vi "Test Pre-arm.vi"() -> ()   [LabVIEW 2021]
uses:
  Instruments/Lockin Digitizer Driver/Lockin Digitizer Configuration.ctl
  DAQmx Lockin Digitizer Driver.lvclass
  C:/GitHub/NHMFL_Core/Libraries/Instruments/Pulse Driver/Lockin Digitizer Driver/Lockin Digitizer Driver.lvclass
panel:
  out "error out":errorcluster
  out "DAQmx Lockin Digitizer Driver out":refnum<class "DAQmx Lockin Digitizer Driver.lvclass">
  in  "DAQmx Lockin Digitizer Driver in":refnum<class "DAQmx Lockin Digitizer Driver.lvclass">
  in  "Lockin Digitizer Configuration":T1={"Post-trigger delay"=0.01, "Post-trigger duration"=0.1, "Rate"=1000000.0, "Ranges"=[10.0], "Re-name channels"=["Bdor", "Idot", "V1", "V2", "I1", "I2", "I3"], "Active channels"="0:6", "External\nclock"=FALSE, "Frequencies"=[1.0, 2.0], "Time\nconstant"=1.0, "Output \namplitudes"=[1.0, 3.0], "Input\nchannles"=["2:3", "4:6"]} {"Output \namplitudes" format="%#_6pV"; "Time\nconstant" format="%#_6ps"; "Frequencies" format="%#_6pHz"; "Rate" format="%#_8pHz"; "Post-trigger duration" format="%#_6ps"; "Post-trigger delay" format="%#_6ps"; "Ranges" format="%#_6pV"}
  # "Digitizer config"
  # "Lock-in config"
  # "#0\n\n#1"
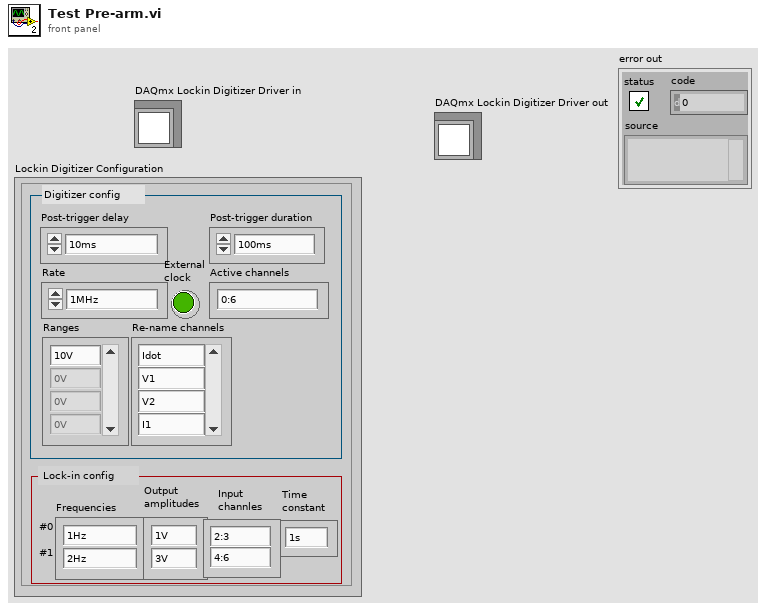
[diagram p1: front panel]
types:
  T1 = typedef "Lockin Digitizer Configuration.ctl" = cluster{"Post-trigger delay":dbl, "Post-trigger duration":dbl, "Rate":dbl, "Ranges":dbl[], "Re-name channels":string[], "Active channels":string, "External\nclock":bool, "Frequencies":dbl[], "Time\nconstant":dbl, "Output \namplitudes":dbl[], "Input\nchannles":string[]}
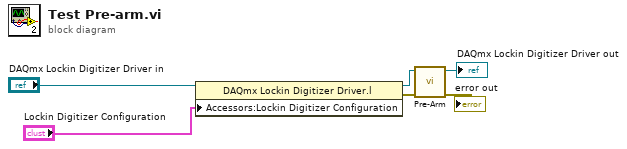
[diagram p0: block diagram]
diagram:
  n1 = property class="DAQmx Lockin Digitizer Driver.l"(reference="DAQmx Lockin Digitizer Driver in", "Accessors:Lockin Digitizer Configuration"="Lockin Digitizer Configuration") -> (reference out=w6:refnum<class "DAQmx Lockin Digitizer Driver.lvclass">, error out=w4:errorcluster)  [unwired: 1 in]
  n2 = call-dynamic "Pre-Arm.vi"("error in (no error)"=w4, "DAQmx Lockin Digitizer Driver in"=w6) -> ("error out"=→"error out":errorcluster, "DAQmx Lockin Digitizer Driver out"=→"DAQmx Lockin Digitizer Driver out":refnum<class "DAQmx Lockin Digitizer Driver.lvclass">)  [unwired: 8 in]
